vi "String Path - Find Folder CHAIN.vi"(0 "String Path":string, 3 "Common Base Path Folder Depth":i32) -> (15 "Relative Parent Folders CHAIN":string[](array[string]), 17 "File Name":string)   [LabVIEW 2022 SP3, in "Generic Utilities.lvclass"]
uses:
  Generic Utilities.lvclass
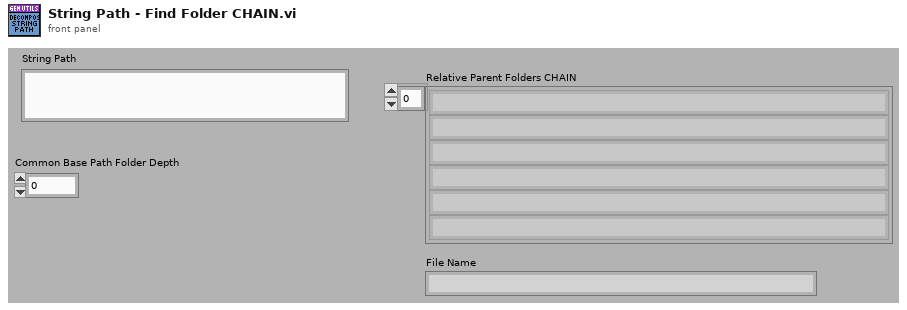
[diagram p1: front panel]
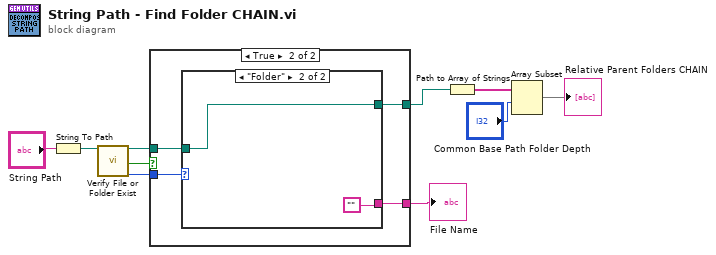
[diagram p0: block diagram]
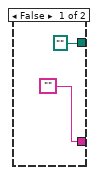
[diagram p2: hidden frame]
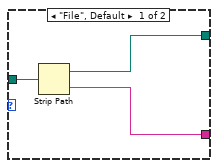
[diagram p3: hidden frame]
diagram:
  n1 = String To Path(string="String Path") -> (path=w4:path)
  n2 = call "Verify File or Folder Exist.vi"("path"=w4) -> ("dup path"=w8:path, "file or folder exists?"=w9:bool, "Path Type"=w7:enum16{"unknown", "File", "Folder"})  [unwired: 16 in]
  n3 = case shown="True" w9 {
    tunnel: ["" w16] -> w10
    tunnel: [path "" w15] -> w3
    tunnel: w8 -> [_ w14]
    tunnel: w7 -> [_ w13]
    frame False {
    }
    frame True {
      n4 = case shown="\"Folder\"" w13 {
        tunnel: [w19 ""] -> w16
        tunnel: [w17 w20] -> w15
        tunnel: w14 -> [w18 w20]
        frame "File", Default {
          n5 = Strip Path(path=w18) -> (stripped path=w17:path, name=w19:string)
        }
        frame "Folder" {
        }
      }
    }
  }
  "File Name" <- w10
  n6 = Path to Array of Strings(0:w3) -> (2:w5:string[])  [unwired: 1 out]
  n7 = Array Subset(array=w5, index="Common Base Path Folder Depth") -> (→"Relative Parent Folders CHAIN":string[])  [unwired: 1 in]
